vi "Suckin.vi"(4 "Abort":refnum<vi>, 6 "Dialog Indicator":refnum<vi>, 7 "Signals":T2, 8 "error in (no error)":errorcluster, 9 "Pressure Controls":T1, 10 "Suction Parameters":refnum<vi>, 11 "Seal Parameters":refnum<vi>) -> (0 "error out":errorcluster, 2 "Minimum Pressure Reached":bool)   [LabVIEW 2012, in "Autopatcher Daemon.lvlib"]
uses:
  Autopatcher Daemon.lvlib
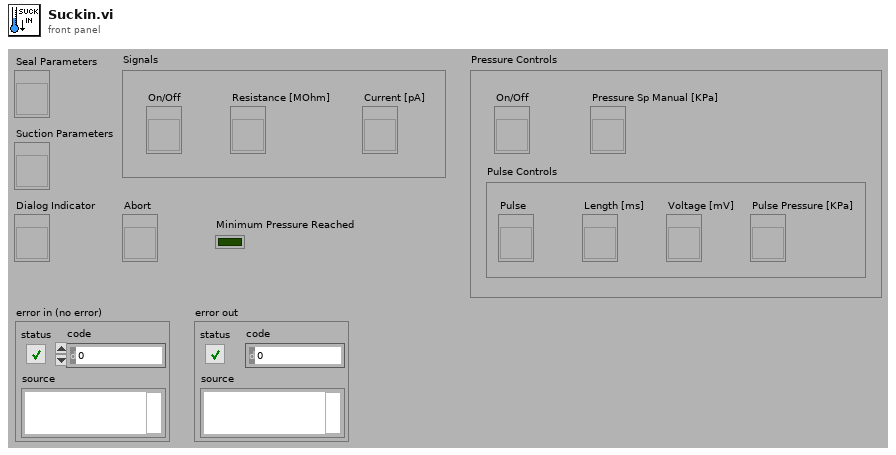
[diagram p1: front panel]
types:
  T1 = cluster{"On/Off":refnum<vi>, "Pulse Controls":cluster{"Pulse":refnum<vi>, "Length [ms]":refnum<vi>, "Voltage [mV]":refnum<vi>, "Pulse Pressure [KPa]":refnum<vi>}, "Pressure Sp Manual [KPa]":refnum<vi>}
  T2 = cluster{"On/Off":refnum<vi>, "Resistance [MOhm]":refnum<vi>, "Current [pA]":refnum<vi>}
  T3 = cluster{"Seal Target [MOhm]":dbl, "Stability Threhsold [%]":dbl, "Seal Timeout [s]":dbl, "Stability Refresh [ms]":dbl}
  T4 = cluster{"Initial Pressure [Kpa]":dbl, "Minimum Pressure [KPa]":dbl, "Decremental Step [KPa]":dbl, "Decremental Threshold [%]":dbl, "Falloff Threshold [%]":dbl, "Falloff Lag [ms]":dbl, "Monitor Refresh [ms]":dbl}
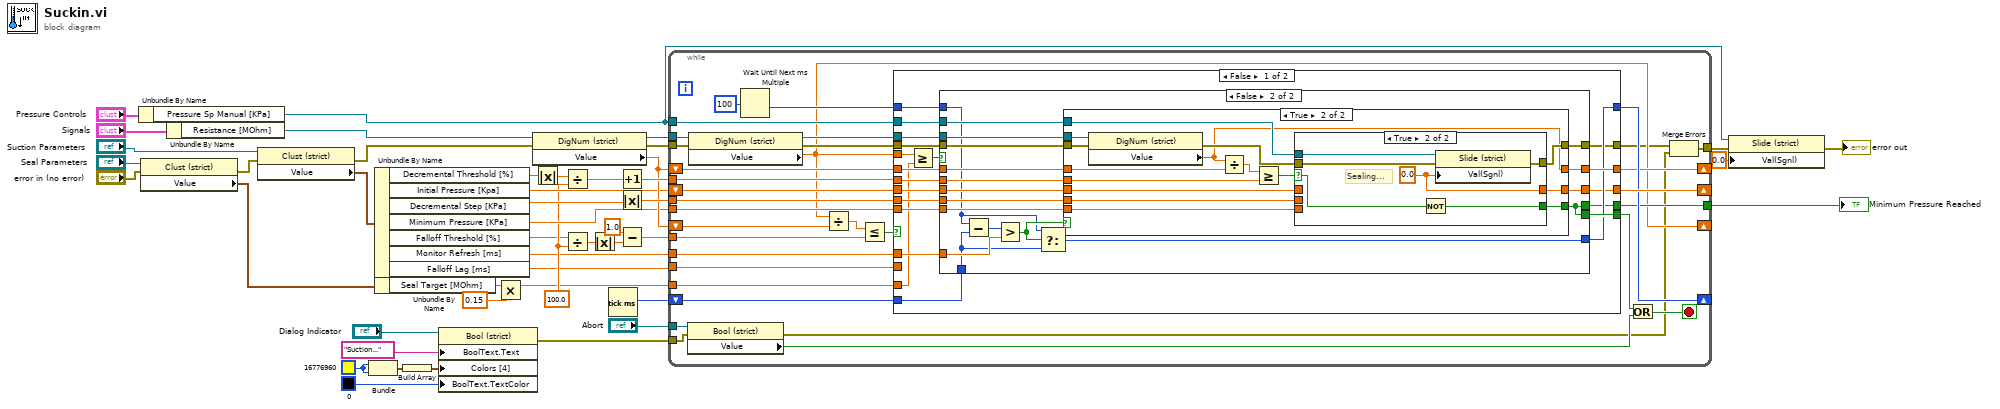
[diagram p0: block diagram]
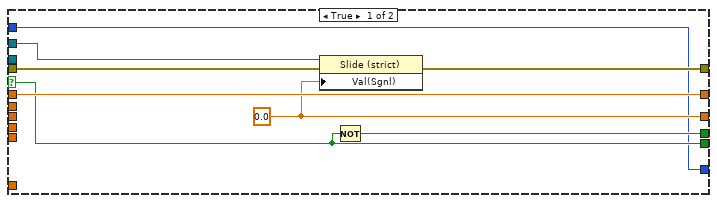
[diagram p2: hidden frame]
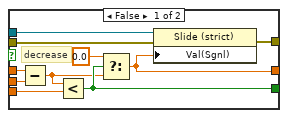
[diagram p4: hidden frame]
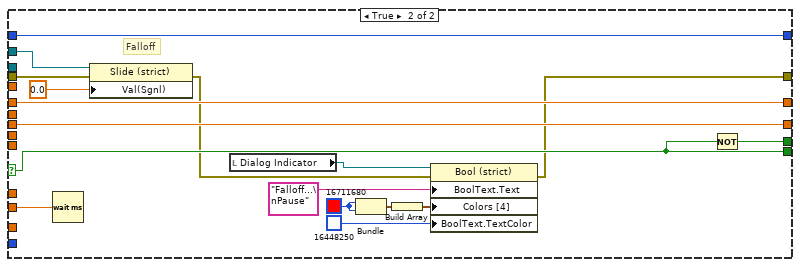
[diagram p5: hidden frame]
diagram:
  w8 = u32 16776960
  w30 = 100.0 ("y")
  n1 = Unbundle By Name("Pressure Controls") -> ("Pressure Sp Manual [KPa]"=w13:refnum<vi>)
  n2 = property class="Clust (strict)"(reference="Seal Parameters", error in="error in (no error)") -> (error out=w20:errorcluster, "Value"=w17:T3)  [unwired: 1 out]
  n3 = Unbundle By Name("Signals") -> ("Resistance [MOhm]"=w34:refnum<vi>)
  n4 = property class="Clust (strict)"(reference="Suction Parameters", error in=w20) -> (error out=w18:errorcluster, "Value"=w22:T4)  [unwired: 1 out]
  n5 = Bundle(w8, w8) -> (w9:cluster{u32, u32})  [unwired: 1 in]
  n6 = Unbundle By Name(w22) -> ("Decremental Threshold [%]"=w2:dbl, "Initial Pressure [Kpa]"=w31:dbl, "Decremental Step [KPa]"=w33:dbl, "Minimum Pressure [KPa]"=w32:dbl, "Falloff Threshold [%]"=w26:dbl, "Monitor Refresh [ms]"=w27:dbl, "Falloff Lag [ms]"=w28:dbl)
  n7 = Unbundle By Name(w17) -> ("Seal Target [MOhm]"=w21:dbl)
  n8 = Build Array(w9) -> (w10:cluster{u32, u32}[])
  n9 = property class="Bool (strict)"(reference="Dialog Indicator", "BoolText.Text"="Suction..." ("Boolean Text.Text"), "Colors [4]"=w10, "BoolText.TextColor"=u32 0) -> (error out=w5:errorcluster)  [unwired: 1 in, 1 out]
  n10 = Multiply(x=w21, y=0.15) -> (x*y=w4:dbl)
  n11 = property class="DigNum (strict)"(reference=w34, error in=w18) -> (reference out=w35:refnum<vi>, error out=w29:errorcluster, "Value"=w36:dbl)
  n12 = Absolute Value(x=w2) -> (abs(x)=w1:dbl)
  n13 = Divide(x=w1, y=w30) -> (x/y=w45:dbl)
  n14 = Divide(x=w26, y=w30) -> (x/y=w38:dbl)
  n15 = Absolute Value(x=w38) -> (abs(x)=w39:dbl)
  n16 = Tick Count (ms)() -> (millisecond timer value=w40:u32)
  n17 = Increment(x=w45) -> (x+1=w43:dbl)
  n18 = Absolute Value(x=w33) -> (abs(x)=w42:dbl)
  n19 = Subtract(x=1.0, y=w39) -> (x-y=w44:dbl)
  n20 = while {
    shift-right: [w52] -> _
    shift-left: w36 -> [w72]
    tunnel: w44 -> [w79]
    tunnel: w43 -> [w76]
    shift-right: [w70] -> _
    shift-left: w31 -> [w75]
    tunnel: w42 -> [w74]
    tunnel: w32 -> [w73]
    tunnel: [w62] -> w41
    shift-right: [w67] -> _
    shift-left: w40 -> [w68]
    tunnel: w27 -> [w69]
    shift-right: [w64] -> _
    shift-left: w36 -> [w65]
    tunnel: w28 -> [w63]
    tunnel: "Abort" -> [w58]
    tunnel: w35 -> [w57]
    tunnel: w13 -> [w56]
    tunnel: w29 -> [w53]
    tunnel: w4 -> [w51]
    tunnel: [w48] -> w15
    tunnel: w5 -> [w47]
    stop <- w60 stop-if-true
    n21 = property class="Bool (strict)"(reference=w58, error in=w47) -> (error out=w49:errorcluster, "Value"=w59:bool)  [unwired: 1 out]
    n22 = property class="DigNum (strict)"(reference=w57, error in=w53) -> (reference out=w55:refnum<vi>, error out=w54:errorcluster, "Value"=w52:dbl)
    n23 = Wait Until Next ms Multiple(millisecond multiple=u32 100) -> (millisecond timer value=w66:u32)
    n24 = Divide(x=w52, y=w72) -> (x/y=w77:dbl)
    n25 = Less Or Equal?(x=w77, y=w79) -> (x <= y?=w78:bool)
    n26 = case shown="False" w78 {
      selector: w78 -> [_ w171]
      tunnel: w76 -> [w93 _]
      tunnel: w75 -> [w99 w177]
      tunnel: w74 -> [w98 _]
      tunnel: w73 -> [w97 _]
      tunnel: [w88 w177] -> w70
      tunnel: [w89 w170] -> w62
      tunnel: w69 -> [w92 _]
      tunnel: w66 -> [w86 w169]
      tunnel: w68 -> [w96 _]
      tunnel: [w90 w169] -> w67
      tunnel: w65 -> [w95 w176]
      tunnel: [w94 w176] -> w64
      tunnel: w63 -> [_ w175]
      tunnel: [w91 w171] -> w61
      tunnel: w52 -> [w80 _]
      tunnel: w56 -> [w85 w173]
      tunnel: w55 -> [w84 _]
      tunnel: w54 -> [w83 w172]
      tunnel: [w82 w162] -> w50
      tunnel: w51 -> [w81 _]
      frame False {
        n27 = Greater Or Equal?(x=w80, y=w81) -> (x >= y?=w87:bool)
        n28 = case shown="False" w87 {
          selector: w87 -> [w102 _]
          tunnel: w99 -> [_ w125]
          tunnel: w98 -> [_ w124]
          tunnel: w97 -> [_ w123]
          tunnel: w96 -> [_ w108]
          tunnel: w95 -> [w107 w122]
          tunnel: [w107 w121] -> w94
          tunnel: w93 -> [_ w120]
          tunnel: w92 -> [_ w109]
          tunnel: [w102 w114] -> w91
          tunnel: [w100 w119] -> w90
          tunnel: w86 -> [w100 w111]
          tunnel: [w101 w114] -> w89
          tunnel: [w106 w118] -> w88
          tunnel: w85 -> [w105 w116]
          tunnel: w84 -> [_ w115]
          tunnel: w83 -> [w104 w113]
          tunnel: [w103 w112] -> w82
          frame True {
            w106 = 0.0 ("Pressure Set Point")
            n29 = property class="Slide (strict)"(reference=w105, error in=w104, "Val(Sgnl)"=w106) -> (error out=w103:errorcluster)  [unwired: 1 out]
            n30 = Not(x=w102) -> (.not. x?=w101:bool)
          }
          frame False {
            n31 = Subtract(x=w111, y=w108) -> (x-y=w110:u32)
            n32 = Greater?(x=w110, y=w109) -> (0:w117:bool)
            n33 = Select(t=w111, s=w117, f=w108) -> (s? t:f=w119:u32)
            n34 = case shown="True" w117 {
              selector: w117 -> [w126 _]
              tunnel: w125 -> [w129 w144]
              tunnel: w124 -> [_ w143]
              tunnel: w123 -> [_ w142]
              tunnel: [w129 w141] -> w118
              tunnel: [w126 w134] -> w114
              tunnel: w122 -> [w128 w138]
              tunnel: w120 -> [_ w140]
              tunnel: [w128 w130] -> w121
              tunnel: w116 -> [_ w136]
              tunnel: w115 -> [_ w135]
              tunnel: w113 -> [w127 w132]
              tunnel: [w127 w131] -> w112
              frame False {
              }
              frame True {
                n35 = property class="DigNum (strict)"(reference=w135, error in=w132) -> (error out=w133:errorcluster, "Value"=w130:dbl)  [unwired: 1 out]
                n36 = Divide(x=w130, y=w138) -> (x/y=w137:dbl)
                n37 = Greater Or Equal?(x=w137, y=w140) -> (x >= y?=w139:bool)
                n38 = case shown="True" w139 {
                  selector: w139 -> [_ w160]
                  tunnel: [w151 w155] -> w141
                  tunnel: w144 -> [w154 _]
                  tunnel: w143 -> [w153 _]
                  tunnel: w142 -> [w152 _]
                  tunnel: [w150 w159] -> w134
                  tunnel: w136 -> [w147 w156]
                  tunnel: w133 -> [w146 w157]
                  tunnel: [w145 w158] -> w131
                  frame False {
                    # "decrease"
                    n39 = Subtract(x=w154, y=w153) -> (x-y=w149:dbl)
                    n40 = Less?(x=w149, y=w152) -> (x < y?=w150:bool)
                    n41 = Select(t=0.0, s=w150, f=w149) -> (s? t:f=w151:dbl)
                    n42 = property class="Slide (strict)"(reference=w147, error in=w146, "Val(Sgnl)"=w151) -> (error out=w145:errorcluster)  [unwired: 1 out]
                  }
                  frame True {
                    w155 = 0.0 ("Value (Signaling)")
                    # "Sealing..."
                    n43 = Not(x=w160) -> (.not. x?=w159:bool)
                    n44 = property class="Slide (strict)"(reference=w156, error in=w157, "Val(Sgnl)"=w155) -> (error out=w158:errorcluster)  [unwired: 1 out]
                  }
                }
              }
            }
          }
        }
      }
      frame True {
        w167 = u32 16711680
        # "Falloff"
        n45 = Wait (ms)(milliseconds to wait=w175) -> ()  [unwired: 1 out]
        n46 = property class="Slide (strict)"(reference=w173, error in=w172, "Val(Sgnl)"=0.0 ("f")) -> (error out=w163:errorcluster)  [unwired: 1 out]
        n47 = local read "Dialog Indicator"() -> (w161:refnum<vi>)
        n48 = Bundle(w167, w167) -> (w166:cluster{u32, u32})  [unwired: 1 in]
        n49 = Build Array(w166) -> (w165:cluster{u32, u32}[])
        n50 = property class="Bool (strict)"(reference=w161, error in=w163, "BoolText.Text"="Falloff...\nPause" ("Boolean Text.Text"), "Colors [4]"=w165, "BoolText.TextColor"=u32 16448250) -> (error out=w162:errorcluster)  [unwired: 1 out]
        n51 = Not(x=w171) -> (.not. x?=w170:bool)
      }
    }
    n52 = Or(x=w61, y=w59) -> (x .or. y?=w60:bool)
    n53 = Merge Errors(w50, w49) -> (w48:errorcluster)
  }
  "Minimum Pressure Reached" <- w41
  n54 = property class="Slide (strict)"(reference=w13, error in=w15, "Val(Sgnl)"=0.0 ("Value")) -> (error out=→"error out":errorcluster)  [unwired: 1 out]
